vi "Constant Query.vi"(8 "error in (no error)":errorcluster, 10 "Model in":refnum<class "Model.lvclass">, 11 "Manual State in":refnum<class "Manual State.lvclass">) -> (0 "error out":errorcluster, 2 "Model out":refnum<class "Model.lvclass">, 3 "Manual State out":refnum<class "Manual State.lvclass">)   [LabVIEW 2016, in "Manual State.lvclass"]
uses:
  Manual State.lvclass
  Model/Model/Model.lvclass
  <vilib>/Platform/TimedLoop/XDataNode/timing_clust.ctl
  <vilib>/Platform/TimedLoop/XDataNode/nitl_modes.ctl
  <vilib>/Platform/TimedLoop/XDataNode/wakeup.ctl
  Globals.vi
  <vilib>/platform/TimedLoop/XDataNode/XDataNode.xnode
  Model/Boot Loader/Boot Loader.lvclass
  <vilib>/Platform/TimedLoop/XDataNode/XDNodeRunTimeDep.lvlib
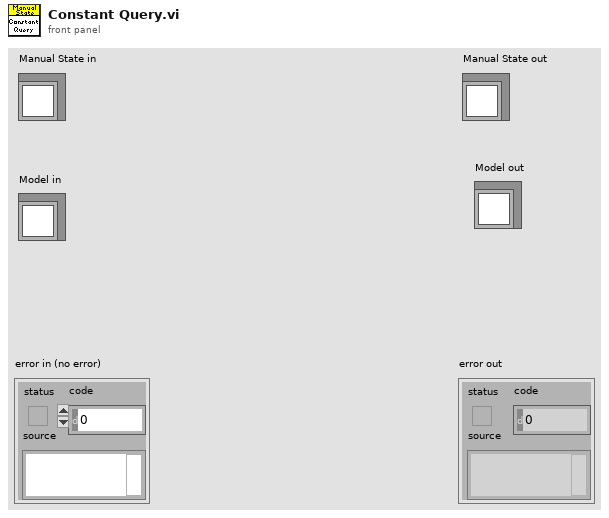
[diagram p1: front panel]
types:
  T1 = typedef "XDNodeRunTimeDep.lvlib/timing_clust.ctl" = cluster{"Expected End [f-1]":u64, "Actual End [f-1]":u64, "Finished Late? [f-1]":bool, "Expected End [i-1]":u64, "Actual End [i-1]":u64, "Finished Late? [i-1]":bool, "Expected Start [i]":u64, "Actual Start [i]":u64, "Expected Start [f]":u64, "Actual Start [f]":u64, "Source Name":string, "Structure Name":string, "Period":i64, "Deadline":i64, "Offset":i64, "Start":i64, "Priority":i32, "Timeout":i32, "Mode":T2, "Wakeup Reason":T3, "Error":errorcluster, "Source Type":string, "Secondary Source Type":string, "Global End Time":u64, "Global Start Time":u64, "Frame Duration":u64, "Iteration Duration":u64, "Assigned CPU":i32, "I/O Scan Engine Mode":u32}
  T2 = typedef "XDNodeRunTimeDep.lvlib/nitl_modes.ctl" = enum32{"No Change", "Process missed periods, maintain original phase", "Discard missed periods, maintain original phase", "Process missed periods, ignore original phase", "Discard missed periods, ignore original phase"}
  T3 = typedef "XDNodeRunTimeDep.lvlib/wakeup.ctl" = enum32{"Normal", "Aborted", "Asynchronous wakeup", "Timing source error", "Timed loop error", "Timeout"}
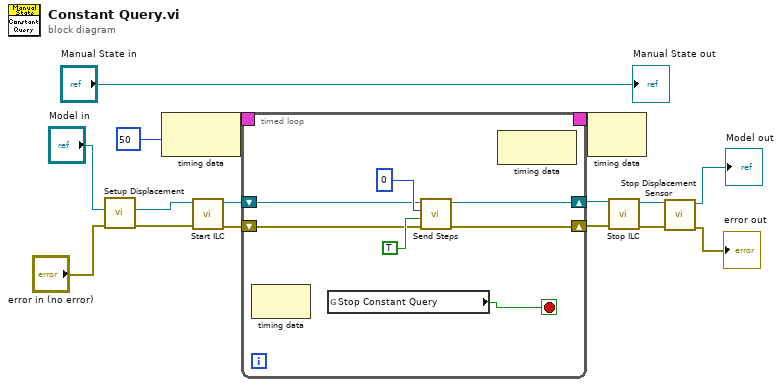
[diagram p0: block diagram]
diagram:
  n1 = call "Setup Displacement.vi"("error in (no error)"="error in (no error)", "Model in"="Model in") -> ("error out"=w14:errorcluster, "Model out"=w15:refnum<class "Model.lvclass">)  [unwired: 7 in, 1 out]
  n2 = node-c288(i64 50) -> (w3:T1)
  n3 = call "Start ILC.vi"("error in (no error)"=w14, "Model in"=w15) -> ("error out"=w10:errorcluster, "Model out"=w11:refnum<class "Model.lvclass">)  [unwired: 8 in]
  n4 = timed-loop {
    shift-right: [w19] -> w5
    shift-left: w11 -> [w21]
    shift-right: [w18] -> w4
    shift-left: w10 -> [w20]
    timing: w3 -> [_]
    timing-out: [_] -> w2
    stop <- w17 stop-if-true
    n5 = node-c288() -> ()  [unwired: 1 in, 1 out]
    n6 = global read "Globals.vi" "Stop Constant Query"() -> (w17:bool)
    n7 = call "Send Steps.vi"("error in (no error)"=w20, "Write Data?"=TRUE, "Command.Steps"=0, "Model in"=w21) -> ("error out"=w18:errorcluster, "Model out"=w19:refnum<class "Model.lvclass">)  [unwired: 6 in]
    n8 = node-c288() -> ()  [unwired: 1 in, 1 out]
  }
  n9 = node-c288(w2) -> ()  [unwired: 1 out]
  n10 = call "Stop ILC.vi"("error in (no error)"=w4, "Model in"=w5) -> ("error out"=w9:errorcluster, "Model out"=w8:refnum<class "Model.lvclass">)  [unwired: 8 in]
  n11 = call "Stop Displacement Sensor.vi"("error in (no error)"=w9, "Model in"=w8) -> ("error out"=→"error out":errorcluster, "Model out"=→"Model out":refnum<class "Model.lvclass">)  [unwired: 8 in]
  "Manual State out" <- "Manual State in"
